vi "Initialize.vi"(8 "error in (no error)":errorcluster, 11 "Thread User Interface in":refnum<class "Thread User Interface.lvclass">) -> (0 "error out":errorcluster, 3 "Thread User Interface out":refnum<class "Thread User Interface.lvclass">)   [LabVIEW 2017, in "PXImc.lvlib" / "Thread User Interface.lvclass"]
uses:
  Thread User Interface.lvclass
  DSF Core.lvlibp/Classes/User Interface/User Interface.lvclass
  Configurations/Thread/Thread Configuration.lvclass
  C:/Git/DSF/Components/DSF Core.lvlibp/Classes/Configuration/Configuration.lvclass
  C:/Git/DSF/Components/DSF Core.lvlibp/Classes/User Interface/User Interface.lvclass
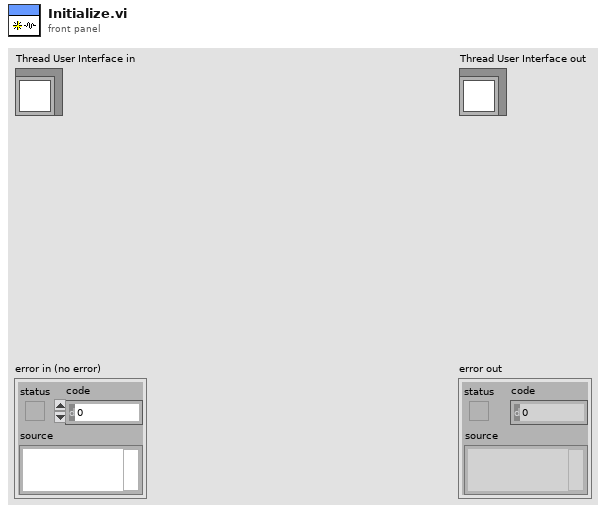
[diagram p1: front panel]
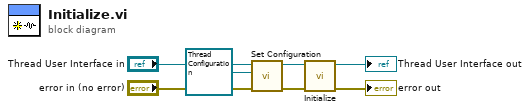
[diagram p0: block diagram]
diagram:
  n1 = call "Set Configuration.vi"("error in (no error)"="error in (no error)", "configuration"=refnum<class "Thread Configuration.lvclass"> refnum ("PXImc.lvlib:PXImc Thread Configuration"), "User Interface in"="Thread User Interface in") -> ("error out"=w2:errorcluster, "User Interface out"=w4:refnum<class "Thread User Interface.lvclass">)  [unwired: 7 in]
  n2 = call-parent "Initialize.vi"("error in (no error)"=w2, "User Interface in"=w4) -> ("error out"=→"error out":errorcluster, "User Interface out"=→"Thread User Interface out":refnum<class "Thread User Interface.lvclass">)  [unwired: 8 in]
